vi "waveform to array.vi"(1 "Start Time":dbl, 2 "Temperature":dbl format="%#_13g", 3 "Voltage Data":waveform(dbl)) -> (0 "array":dbl[][](array[numeric]))   [LabVIEW 2017]
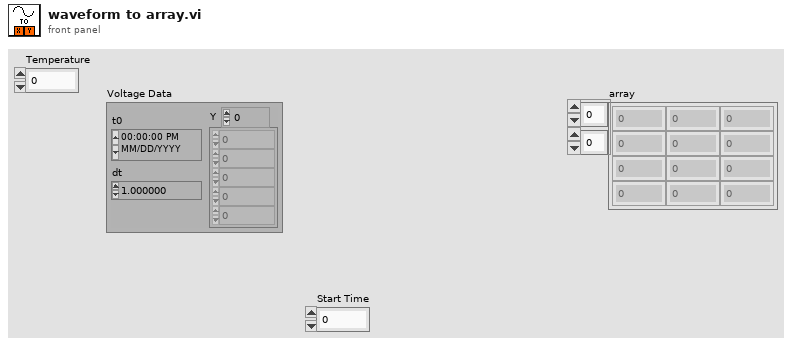
[diagram p1: front panel]
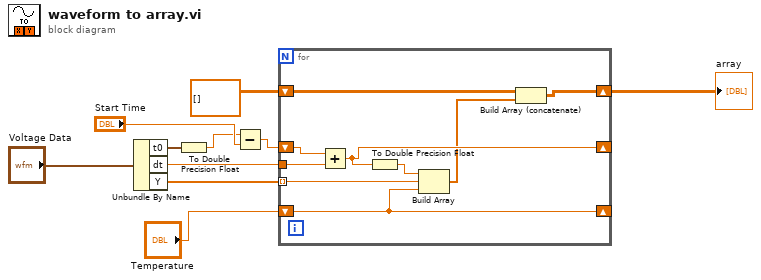
[diagram p0: block diagram]
diagram:
  n1 = Unbundle By Name("Voltage Data") -> ("t0"=w2:timestamp, "dt"=w8:dbl, "Y"=w9:dbl[])
  n2 = To Double Precision Float(number=w2) -> (double precision float=w1:dbl)
  n3 = Subtract(x=w1, y="Start Time") -> (x-y=w5:dbl)
  n4 = for {
    tunnel: w9 -> [w16] mode=indexing
    tunnel: w8 -> [w19]
    shift-right: [w15] -> _
    shift-left: w5 -> [w18]
    shift-right: [w12] -> w6
    shift-left: dbl[][] [] ("appended array") -> [w13]
    shift-right: [w11] -> _
    shift-left: "Temperature" -> [w11]
    n5 = Add(x=w18, y=w19) -> (x+y=w15:dbl)
    n6 = To Double Precision Float(number=w15) -> (double precision float=w17:dbl)
    n7 = Build Array(w17, w16, w11) -> (w14:dbl[])
    n8 = Build Array (concatenate)(w13, w14) -> (w12:dbl[][])
  }
  "array" <- w6
